vi "LINX Serial Benchmark.vi"() -> ()   [LabVIEW 2013]
uses:
  <vilib>/Instr/_visa.llb/VISA Configure Serial Port (Instr).vi
  <vilib>/ptbypt/NI_PtbyPt.lvlib
panel:
  out "Loop Time vs Packet Size - Serial - Arduino Uno":dbl(graph)
  out "Failed Packets":i32
  out "Iteration":i32
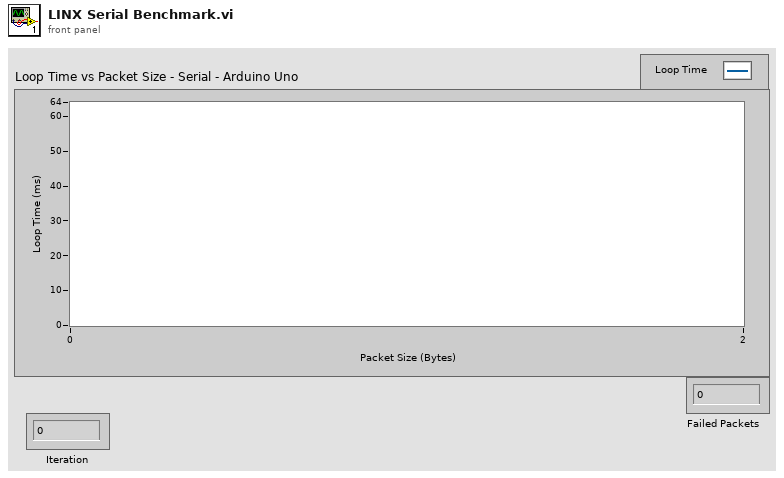
[diagram p1: front panel]
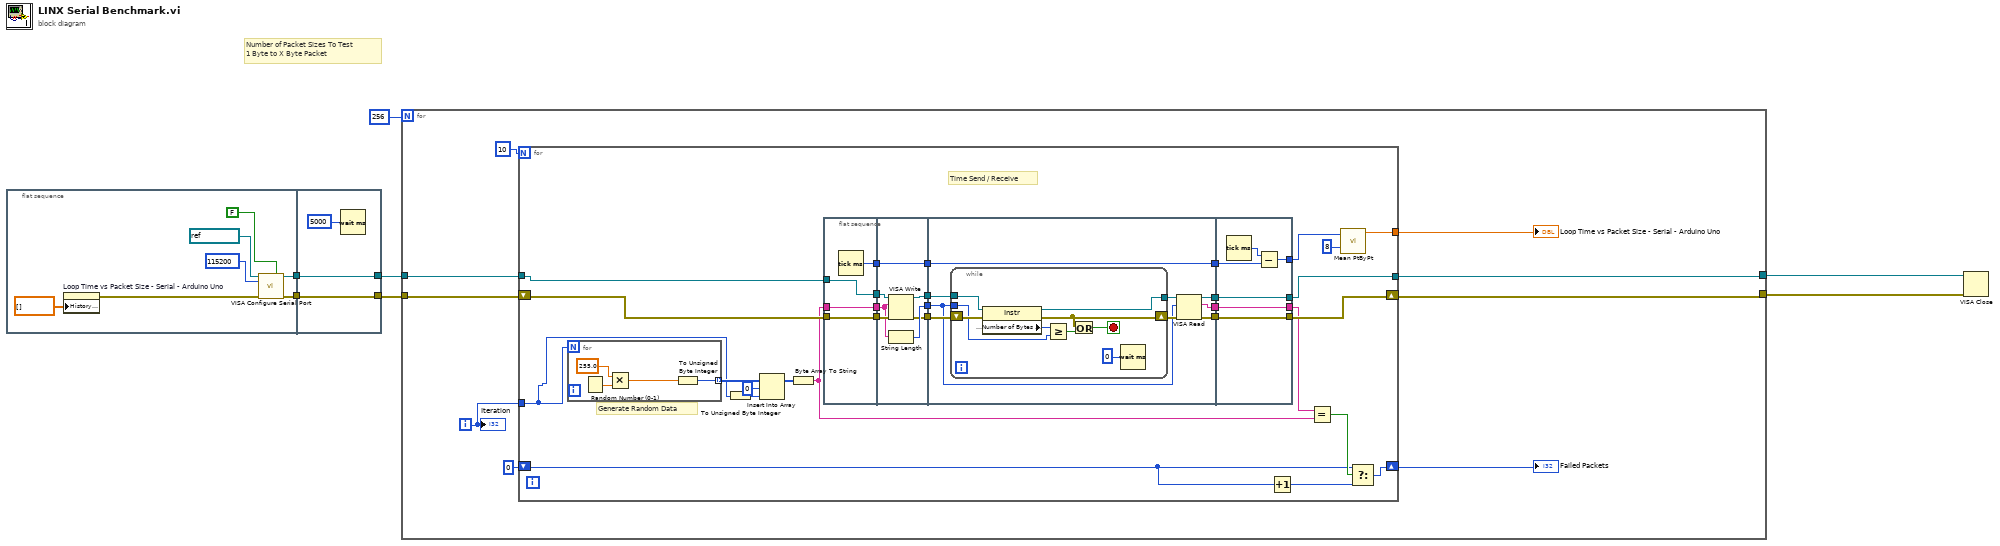
[diagram p0: block diagram]
diagram:
  # "Number of Packet Sizes To Test\n1 Byte to X Byte Packet"
  n1 = flat-sequence {
    tunnel: [w10] -> w5
    tunnel: [w8] -> w3
    tunnel: [w15] -> w6
    tunnel: w5 -> [w15]
    tunnel: [w16] -> w4
    tunnel: w3 -> [w16]
    frame #0 {
      n2 = property on="Loop Time vs Packet Size - Serial - Arduino Uno" class="WFChart (strict)"("History Data"=dbl[] []) -> (error out=w9:errorcluster)  [unwired: 2 in, 1 out]
      n3 = call-poly "VISA Configure Serial Port"("VISA resource name"=refnum<visa-resource-name> "COM9", "Enable Termination\nChar (T)"=FALSE ("Enable Termination\nChar (T)"), "baud rate (9600)"=u32 115200, "error in (no error)"=w9) -> ("VISA resource name out"=w8:refnum<visa-resource-name>, "error out"=w10:errorcluster)  [unwired: 10 in]
    }
    frame #1 {
      n4 = Wait (ms)(milliseconds to wait=u32 5000) -> ()  [unwired: 1 out]
    }
  }
  n5 = for {
    N: 256 -> [_]
    tunnel: w6 -> [w21]
    tunnel: w4 -> [w22]
    tunnel: [w20] -> w2
    tunnel: [w19] -> w1
    i -> [w18]
    n6 = for {
      N: 10 -> [_]
      shift-right: [w51] -> w19
      shift-left: w21 -> [w33]
      tunnel: [w46] -> w20
      shift-right: [w37] -> w25
      shift-left: 0 -> [w38]
      tunnel: [w36] -> w24
      tunnel: w22 -> [w34]
      tunnel: w18 -> [w28]
      # "Time Send / Receive"
      # "Generate Random Data"
      n7 = for {
        N: w28 -> [_]
        tunnel: [w57] -> w31 mode=indexing
        n8 = Random Number (0-1)() -> (number: 0 to 1=w60:dbl)
        n9 = Multiply(x=255.0, y=w60) -> (x*y=w58:dbl)
        n10 = To Unsigned Byte Integer(number=w58) -> (unsigned 8bit integer=w57:u8)
      }
      n11 = To Unsigned Byte Integer(number=w28) -> (unsigned 8bit integer=w30:u8)
      n12 = Insert Into Array(array=w31, index=0, new element=w30) -> (w29:u8[])
      n13 = Byte Array To String(unsigned byte array=w29) -> (string=w32:string)
      n14 = flat-sequence {
        tunnel: w33 -> [w64]
        tunnel: [w64] -> w53
        tunnel: [w63] -> w50
        tunnel: [w62] -> w43
        tunnel: w32 -> [w62]
        tunnel: [w61] -> w35
        tunnel: w34 -> [w61]
        tunnel: [w66] -> w56
        tunnel: [w69] -> w55
        tunnel: [w71] -> w54
        tunnel: w53 -> [w68]
        tunnel: w50 -> [w70]
        tunnel: [w70] -> w49
        tunnel: w43 -> [w67]
        tunnel: w35 -> [w65]
        tunnel: w56 -> [w74]
        tunnel: w55 -> [w76]
        tunnel: w54 -> [w72]
        tunnel: [w79] -> w52
        tunnel: w49 -> [w80]
        tunnel: [w80] -> w48
        tunnel: [w78] -> w47
        tunnel: [w77] -> w41
        tunnel: [w95] -> w51
        tunnel: w52 -> [w95]
        tunnel: w48 -> [w93]
        tunnel: w47 -> [w92]
        tunnel: [w92] -> w46
        tunnel: [w91] -> w45
        tunnel: [w90] -> w42
        tunnel: w41 -> [w90]
        frame #0 {
          n15 = Tick Count (ms)() -> (millisecond timer value=w63:u32)
        }
        frame #1 {
          n16 = VISA Write(VISA resource name=w65, write buffer=w67, error in (no error)=w68) -> (VISA resource name out=w66:refnum<visa-resource-name>, error out=w69:errorcluster)  [unwired: 1 out]
          n17 = String Length(string=w67) -> (length=w71:i32)
        }
        frame #2 {
          n18 = while {
            shift-right: [w84] -> w75
            shift-left: w76 -> [w88]
            tunnel: [w87] -> w73
            tunnel: w74 -> [w86]
            tunnel: w72 -> [w81]
            stop <- w82 stop-if-true
            n19 = property class="Instr"(reference=w86, error in=w88) -> (reference out=w87:refnum<visa-resource-name>, error out=w84:errorcluster, "Serial Settings:Number of Bytes at Serial Port"=w85:u32)
            n20 = Greater Or Equal?(x=w85, y=w81) -> (x >= y?=w83:bool)
            n21 = Or(x=w84, y=w83) -> (x .or. y?=w82:bool)
            n22 = Wait (ms)(milliseconds to wait=u32 0) -> ()  [unwired: 1 out]
          }
          n23 = VISA Read(VISA resource name=w73, byte count=w72, error in (no error)=w75) -> (VISA resource name out=w78:refnum<visa-resource-name>, read buffer=w77:string, error out=w79:errorcluster)  [unwired: 1 out]
        }
        frame #3 {
          n24 = Tick Count (ms)() -> (millisecond timer value=w94:u32)
          n25 = Subtract(x=w94, y=w93) -> (x-y=w91:u32)
        }
      }
      n26 = Increment(x=w38) -> (x+1=w39:i32)
      n27 = Equal?(x=w42, y=w32) -> (x = y?=w40:bool)
      n28 = call <vilib>:"Mean PtByPt.vi"("x"=w45, "sample length"=8) -> ("mean"=w36:dbl)  [unwired: 2 in, 1 out]
      n29 = Select(t=w38, s=w40, f=w39) -> (s? t:f=w37:i32)
    }
    "Failed Packets" <- w25
    "Loop Time vs Packet Size - Serial - Arduino Uno" <- w24
    "Iteration" <- w18
  }
  n30 = VISA Close(VISA resource name=w2, error in (no error)=w1) -> ()  [unwired: 1 out]
